vi "Wait for Network Connections.vi"(8 "error in (no error)":errorcluster, 9 "Handler VI ref":T1, 10 "Ethernet Address":u32, 11 "FPGA Refnum in":T2) -> (0 "error out":errorcluster, 3 "# Network Connections":i32)   [LabVIEW 2020]
doc: "Author: Scott Hannahs <sth@magnet.fsu.edu>\nCopyright 2018 Florida State University, All rights reserved."
uses:
  RT Controls/FPGA SCH Digitizer Ref.ctl
  Net Conn Handler VI.ctl
  RT Host Globals.vi
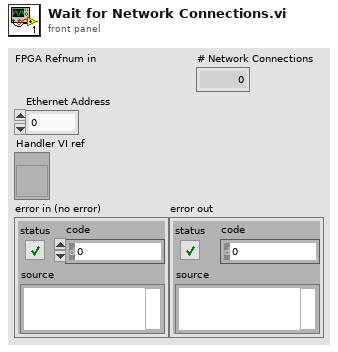
[diagram p1: front panel]
types:
  T1 = typedef "Net Conn Handler VI.ctl" = refnum<vi>
  T2 = typedef "FPGA SCH Digitizer Ref.ctl" = refnum<k20>
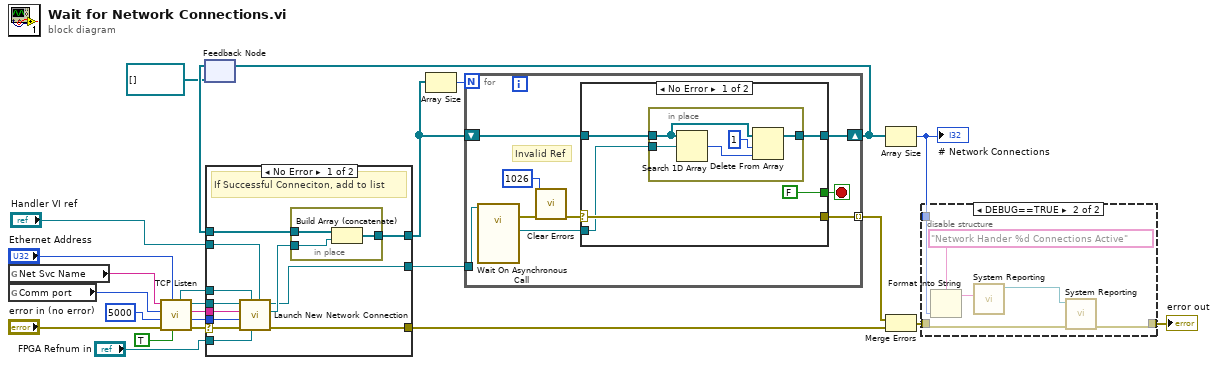
[diagram p0: block diagram]
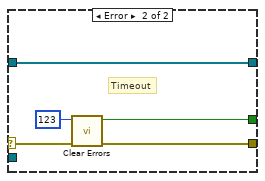
[diagram p3: hidden frame]
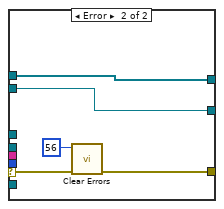
[diagram p4: hidden frame]
diagram:
  n1 = global read "RT Host Globals.vi" "Net Svc Name"() -> (w7:string)
  n2 = global read "RT Host Globals.vi" "Comm port"() -> (w23:u16)
  n3 = call <vilib>:"TCP Listen.vi"("resolve remote address (T)"=TRUE, "net address"="Ethernet Address", "error in (no error)"="error in (no error)", "timeout ms (wait forever: -1)"=5000, "port"=w23, "service name"=w7) -> ("error out"=w20:errorcluster, "remote port"=w16:u16, "remote address"=w18:string, "connection ID"=w15:refnum<k5>, "listener ID"=w14:refnum<k5>)  [unwired: 1 in]
  n4 = feedback #1(refnum<k5>[] []) -> (w13:refnum<k5>[])
  n5 = case shown="No Error" w20 {
    selector: w20 -> [w36 w42]
    tunnel: w14 -> [w35 _]
    tunnel: w15 -> [w34 _]
    tunnel: w16 -> [w32 _]
    tunnel: w18 -> [w33 _]
    tunnel: [w28 w43] -> w10
    tunnel: "FPGA Refnum in" -> [w31 _]
    tunnel: [w30 w41] -> w2
    tunnel: w13 -> [w29 w41]
    tunnel: "Handler VI ref" -> [w27 w40]
    tunnel: [w25 w40] -> w4
    frame No Error {
      # "If Successful Conneciton, add to list"
      n6 = call "Launch New Network Connection.vi"("Handler VI ref"=w27, "FPGA Ref"=w31, "Listener ID"=w35, "error in (no error)"=w36, "Remote Port"=w32, "Remote Address"=w33, "Connection ID"=w34) -> ("error out"=w28:errorcluster, "conn ID Out"=w26:refnum<k5>, "Handler VI Ref out"=w25:T1)  [unwired: 2 in]
      n7 = in-place {
        in-place-border: w26 -> [w39]
        in-place-border: [w38] -> w30
        in-place-border: w29 -> [w37]
        n8 = Build Array (concatenate)(w37, w39) -> (w38:refnum<k5>[])
      }
    }
    frame Error {
      n9 = call <vilib>:"Clear Errors.vi"("error in (no error)"=w42, "specific error code to clear (0: all)"=56) -> ("error out"=w43:errorcluster)  [unwired: 4 in, 1 out]
    }
  }
  n10 = Array Size(array=w2) -> (size(s)=w3:i32)
  n11 = for {
    N: w3 -> [_]
    tunnel: [w51] -> w11 mode=indexing
    shift-right: [w52] -> w12
    shift-left: w2 -> [w53]
    tunnel: w4 -> [w46]
    stop <- w45 stop-if-true
    # "Invalid Ref"
    n12 = call-by-ref "Wait On Asynchronous Call"(reference=w46) -> (error out=w49:errorcluster, "connection ID out"=w47:refnum<k5>)  [unwired: 11 in, 2 out]
    n13 = call <vilib>:"Clear Errors.vi"("error in (no error)"=w49, "specific error code to clear (0: all)"=1026) -> ("error out"=w48:errorcluster)  [unwired: 4 in, 1 out]
    n14 = case shown="No Error" w48 {
      selector: w48 -> [w56 w66]
      tunnel: w53 -> [w58 w68]
      tunnel: [w57 w68] -> w52
      tunnel: [w56 w65] -> w51
      tunnel: w47 -> [w55 _]
      tunnel: [FALSE ("specific error cleared?") w64] -> w45
      frame No Error {
        n15 = in-place {
          in-place-border: w55 -> [w63]
          in-place-border: w58 -> [w60]
          in-place-border: [w59] -> w57
          n16 = Search 1D Array(1D array=w60, element=w63) -> (index of element=w61:i32)  [unwired: 1 in]
          n17 = Delete From Array(array=w60, length=1, index=w61) -> (array with subset deleted=w59:refnum<k5>[])  [unwired: 1 out]
        }
      }
      frame Error {
        # "Timeout"
        n18 = call <vilib>:"Clear Errors.vi"("error in (no error)"=w66, "specific error code to clear (0: all)"=123) -> ("error out"=w65:errorcluster, "specific error cleared?"=w64:bool)  [unwired: 4 in]
      }
    }
  }
  n19 = feedback-in #1(w12) -> ()
  n20 = Array Size(array=w12) -> (size(s)=w1:i32)
  "# Network Connections" <- w1
  n21 = Merge Errors(w11, w10) -> (w9:errorcluster)
  n22 = disable-structure shown="DEBUG==TRUE" {
    disable-tunnel: w9 -> [w69 w75]
    disable-tunnel: [w69 w74] -> w8
    disable-tunnel: w1 -> [_ w71]
    frame condition #0 (active) {
    }
    frame condition #1 {
      n23 = Format Into String(format string="Network Hander %d Connections Active", w71) -> (resulting string=w70:string)  [unwired: 2 in, 1 out]
      n24 = call "System Reporting.vi"("String"=w70) -> ("Byte Stream File out"=w73:refnum<file>)  [unwired: 9 in, 1 out]
      n25 = call "System Reporting.vi"("Error In"=w75, "Byte Stream File in"=w73) -> ("Error Out"=w74:errorcluster)  [unwired: 8 in, 1 out]
    }
  }
  "error out" <- w8
